vi "Create TDMS Channels - DAQ AI.vi"(7 "DAQ AI Configuration":T1={"AI Channels"="Dev1/ai0", "Min (V)"=-5.0, "Max (V)"=5.0, "Terminal Config"=-1, "Sample Rate (Hz)"=1000.0, "#Samples"=100} {"Terminal Config" items=["Default"=-1, "RSE"=10083, "NRSE"=10078, "Differential"=10106, "Pseudodifferential"=12529]; "Min (V)" format="%#_13g"; "Max (V)" format="%#_13g"; "Sample Rate (Hz)" format="%#_13g"}, 8 "error in (no error)":errorcluster, 10 "group name in":string="Log", 11 "TDMS ref in":refnum<k34>) -> (0 "error out":errorcluster, 1 "Signal Names":string[](array[string]), 2 "group name out":string="Log", 3 "TDMS ref out":refnum<k34>, 4 "Signal Units":string[](array[string]))   [LabVIEW 2021, in "XNET-CAN-Signal-Logger.lvlib"]
uses:
  XNET-CAN-Signal-Logger.lvlib
  Typedef/Def-DAQ AI Configuration.ctl
  <resource>/objmgr/daqmx.rc
panel:
  in  "AI.Voltage.Units":i32(ring)=10348 items=["Volts"=10348, "From Custom Scale"=10065, "From TEDS"=12516]
  in  "ScaleType":i32(ring)=10447 items=["Linear"=10447, "Map Ranges"=10448, "Polynomial"=10449, "Table"=10450]
  in  "AI.TermCfg":i32(ring)=10083 items=["RSE"=10083, "NRSE"=10078, "Differential"=10106, "Pseudodifferential"=12529]
  in  "BusType":i32(ring)=12582 items=["PCI"=12582, "PCIe"=13612, "PXI"=12583, "PXIe"=14706, "SCXI"=12584, "SCC"=14707, "PCCard"=12585, "USB"=12586, "CompactDAQ"=14637, "CompactRIO"=16143, "TCP/IP"=14828, "Unknown"=12588, "SwitchBlock"=15870]
  in  "ChanType":i32(ring)=10100 items=["Analog Input"=10100, "Analog Output"=10102, "Digital Input"=10151, "Digital Output"=10153, "Counter Input"=10131, "Counter Output"=10132]
  in  "AI.MeasType":i32(ring)=10322 items=["Voltage"=10322, "Voltage RMS"=10350, "Current"=10134, "Current RMS"=10351, "More:Voltage:Custom with Excitation"=10323, "More:Bridge (V/V)"=15908, "Frequency"=10181, "Resistance"=10278, "Temperature:Thermocouple"=10303, "Temperature:Thermistor"=10302, "Temperature:RTD"=10301, "Temperature:Built-in Sensor"=10311, "Strain Gage"=10300, "Rosette Strain Gage"=15980, "Position:LVDT"=10352, "Position:RVDT"=10353, "Position:Eddy Current Proximity Probe"=14835, "Accelerometer"=10356, "Acceleration:Charge"=16104, "Acceleration:4 Wire DC Voltage"=16106, "Velocity:IEPE Sensor"=15966, "Force:Bridge"=15899, "Force:IEPE Sensor"=15895, "Pressure:Bridge"=15902, "Sound Pressure:Microphone"=10354, "Torque:Bridge"=15905, "TEDS Sensor"=12531, "Charge"=16105, "Power"=16201]
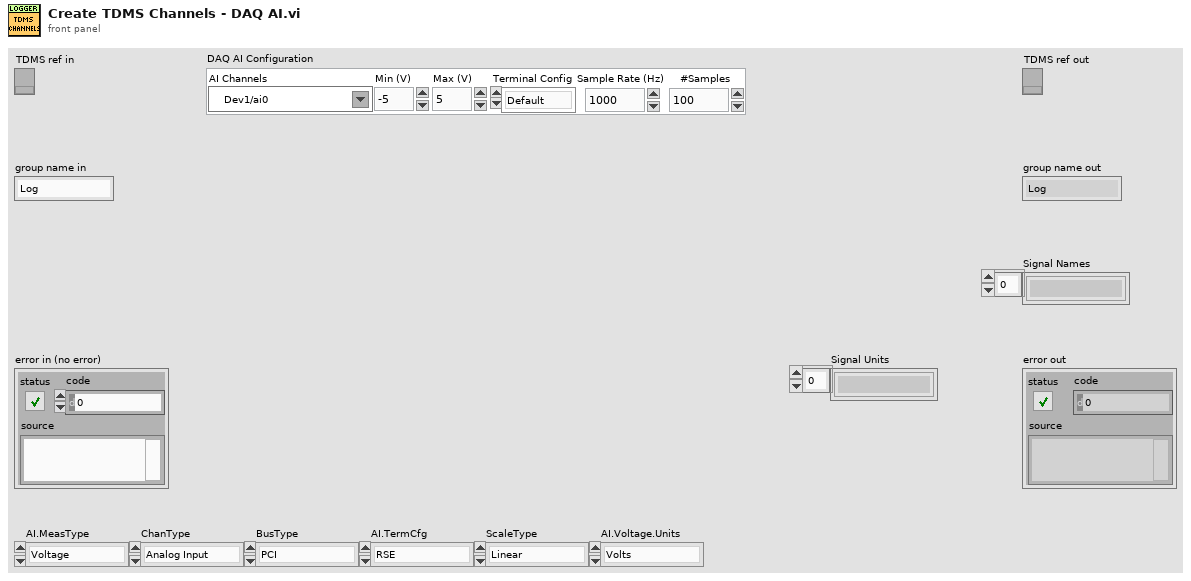
[diagram p1: front panel]
types:
  T1 = typedef "XNET-CAN-Signal-Logger.lvlib/Def-DAQ AI Configuration.ctl" = cluster{"AI Channels":tag, "Min (V)":dbl, "Max (V)":dbl, "Terminal Config":i32, "Sample Rate (Hz)":dbl, "#Samples":i32}
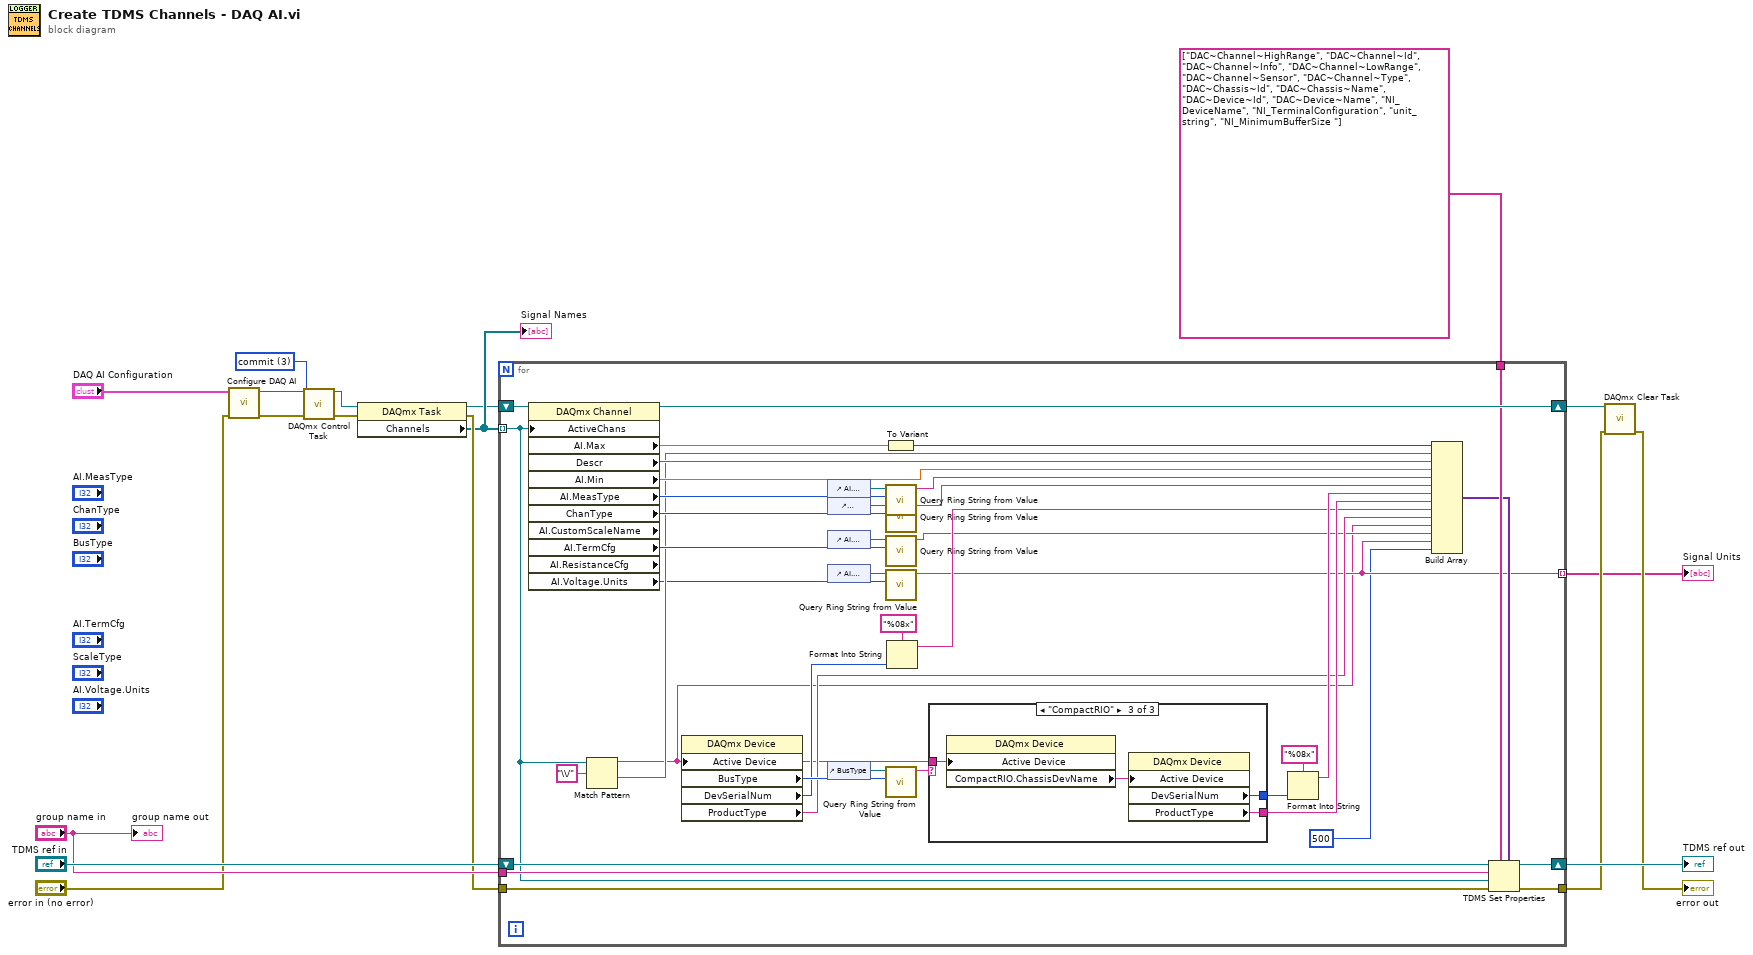
[diagram p0: block diagram]
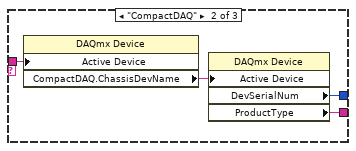
[diagram p3: hidden frame]
diagram:
  w11 = 3 items=["verify"=2, "reserve"=4, "commit"=3, "unreserve"=5, "abort"=6] ("action")
  n1 = call "Configure DAQ AI.vi"("error in"="error in (no error)", "DAQ Configuration"="DAQ AI Configuration") -> ("error out"=w12:errorcluster, "DAQ Task ref out"=w13:refnum<k21>)  [unwired: 8 in]
  n2 = call <vilib>:"DAQmx Control Task.vi"("task/channels in"=w13, "action"=w11, "error in"=w12) -> ("task out"=w9:refnum<k21>, "error out"=w10:errorcluster)  [unwired: 11 in]
  n3 = property class="DAQmx Task"(reference=w9, error in=w10) -> (reference out=w4:refnum<k21>, error out=w6:errorcluster, "Channels"=w5:refnum<k21>[])
  "Signal Names" <- w5
  n4 = for {
    shift-right: [w58] -> w18
    shift-left: "TDMS ref in" -> [w59]
    tunnel: [w57] -> w8
    tunnel: "group name in" -> [w56]
    tunnel: w5 -> [w24] mode=indexing
    tunnel: w6 -> [w55]
    shift-right: [w53] -> w3
    shift-left: w4 -> [w54]
    tunnel: string[] ["DAC~Channel~HighRange", "DAC~Channel~Id", "DAC~Channel~Info", "DAC~Channel~LowRange", "DAC~Channel~Sensor", "DAC~Channel~Type", "DAC~Chassis~Id", "DAC~Chassis~Name", "DAC~Device~Id", "DAC~Device~Name", "NI_DeviceName", "NI_TerminalConfiguration", "unit_string", "NI_MinimumBufferSize "] ("property names") -> [w52]
    tunnel: [w21] -> w1 mode=indexing
    n5 = property class="DAQmx Channel" props=["ActiveChans", "AI.Max", "Descr", "AI.Min", "AI.MeasType", "ChanType", "AI.CustomScaleName", "AI.TermCfg", "AI.ResistanceCfg", "AI.Voltage.Units"](reference=w54, "ActiveChans"=w24) -> (reference out=w53:refnum<k21>, "AI.Max"=w51:dbl, "Descr"=w49:string, "AI.Min"=w48:dbl, "AI.MeasType"=w44:i32, "ChanType"=w42:i32, "AI.TermCfg"=w28:i32, "AI.Voltage.Units"=w22:i32)  [unwired: 1 in, 3 out]
    n6 = Match Pattern(string=w24, regular expression="\\/") -> (before substring=w20:string, after substring=w26:string)  [unwired: 1 in, 2 out]
    n7 = property class="DAQmx Device"("Active Device"=w20) -> ("BusType"=w45:i32, "DevSerialNum"=w34:u32, "ProductType"=w30:string)  [unwired: 2 in, 2 out]
    n8 = control-ref of="AI.MeasType"() -> (w40:refnum<vi>)
    n9 = control-ref of="ChanType"() -> (w39:refnum<vi>)
    n10 = control-ref of="AI.TermCfg"() -> (w29:refnum<vi>)
    n11 = control-ref of="AI.Voltage.Units"() -> (w23:refnum<vi>)
    n12 = control-ref of="BusType"() -> (w46:refnum<vi>)
    n13 = To Variant(anything=w51) -> (Variant=w50:variant)
    n14 = call "Query Ring String from Value.vi"("AI.MeasType"=w44, "Ring Ref"=w40) -> ("String"=w43:string)  [unwired: 8 in, 1 out]
    n15 = call "Query Ring String from Value.vi"("AI.MeasType"=w42, "Ring Ref"=w39) -> ("String"=w41:string)  [unwired: 8 in, 1 out]
    n16 = call "Query Ring String from Value.vi"("AI.MeasType"=w28, "Ring Ref"=w29) -> ("String"=w27:string)  [unwired: 8 in, 1 out]
    n17 = call "Query Ring String from Value.vi"("AI.MeasType"=w22, "Ring Ref"=w23) -> ("String"=w21:string)  [unwired: 8 in, 1 out]
    n18 = call "Query Ring String from Value.vi"("AI.MeasType"=w45, "Ring Ref"=w46) -> ("String"=w38:string)  [unwired: 8 in, 1 out]
    n19 = Format Into String(format string="%08x", w34) -> (resulting string=w31:string)  [unwired: 2 in, 1 out]
    n20 = case shown="\"CompactRIO\"" w38 {
      tunnel: w20 -> [_ w63 w67]
      tunnel: [_ w61 w65] -> w37
      tunnel: [_ w60 w64] -> w32
      frame Default {
      }
      frame "CompactDAQ" {
        n21 = property class="DAQmx Device"("Active Device"=w63) -> ("CompactDAQ.ChassisDevName"=w62:tag)  [unwired: 2 in, 2 out]
        n22 = property class="DAQmx Device"("Active Device"=w62) -> ("DevSerialNum"=w61:u32, "ProductType"=w60:string)  [unwired: 2 in, 2 out]
      }
      frame "CompactRIO" {
        n23 = property class="DAQmx Device"("Active Device"=w67) -> ("CompactRIO.ChassisDevName"=w66:tag)  [unwired: 2 in, 2 out]
        n24 = property class="DAQmx Device"("Active Device"=w66) -> ("DevSerialNum"=w65:u32, "ProductType"=w64:string)  [unwired: 2 in, 2 out]
      }
    }
    n25 = Format Into String(format string="%08x", w37) -> (resulting string=w33:string)  [unwired: 2 in, 1 out]
    n26 = Build Array(w50, w26, w49, w48, w43, w41, w33, w32, w31, w30, w20, w27, w21, u32 500 ("Start Bit")) -> (w25:variant[])
    n27 = TDMS Set Properties(5:w25, 7:w52, 8:w55, 9:w24, 10:w56, 11:w59) -> (0:w57:errorcluster, 3:w58:refnum<k34>)  [unwired: 2 out]
  }
  "TDMS ref out" <- w18
  "Signal Units" <- w1
  n28 = call <vilib>:"DAQmx Clear Task.vi"("task in"=w3, "error in"=w8) -> ("error out"=→"error out":errorcluster)  [unwired: 13 in]
  "group name out" <- "group name in"
